vi "InitCurrentSource.vi"(2 "error out 2":errorcluster, 3 "reference out 2":refnum<visa-resource-name>) -> (0 "error out":errorcluster, 1 "reference out":refnum<visa-resource-name>)   [LabVIEW 2009]
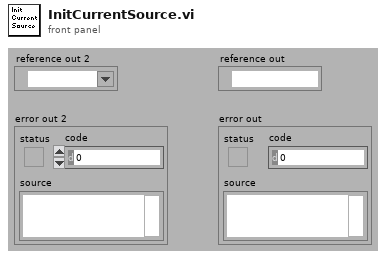
[diagram p1: front panel]
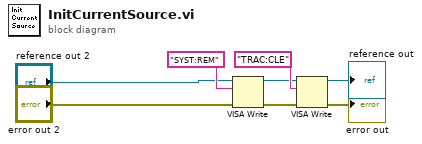
[diagram p0: block diagram]
diagram:
  n1 = VISA Write(VISA resource name="reference out 2", write buffer="SYST:REM", error in (no error)="error out 2") -> (VISA resource name out=w4:refnum<visa-resource-name>, error out=w5:errorcluster)  [unwired: 1 out]
  n2 = VISA Write(VISA resource name=w4, write buffer="TRAC:CLE", error in (no error)=w5) -> (VISA resource name out=→"reference out":refnum<visa-resource-name>, error out=→"error out":errorcluster)  [unwired: 1 out]
